vi "Read Friction Coefficient.vi"(8 "error in":errorcluster, 11 "Friction in":refnum<class "Friction.lvclass">) -> (0 "error out":errorcluster, 2 "Friction Coefficient":dbl, 3 "Friction out":refnum<class "Friction.lvclass">)   [LabVIEW 2016, in "Friction.lvclass"]
uses:
  Friction.lvclass
  Friction.lvclass/Friction.ctl
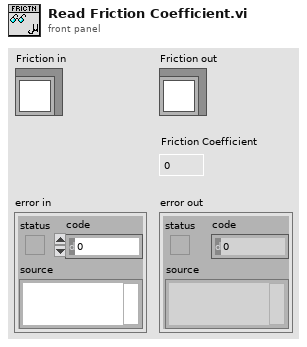
[diagram p1: front panel]
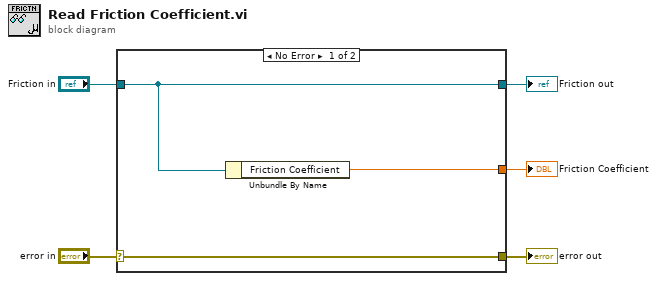
[diagram p0: block diagram]
diagram:
  n1 = case shown="No Error" "error in" {
    selector: "error in" -> [w8 w9]
    tunnel: [w8 w9] -> w4
    tunnel: [w7 w10] -> w2
    tunnel: "Friction in" -> [w7 w10]
    tunnel: [w6 _] -> w1
    frame No Error {
      n2 = Unbundle By Name(w7) -> ("Friction Coefficient"=w6:dbl)
    }
    frame Error {
    }
  }
  "error out" <- w4
  "Friction out" <- w2
  "Friction Coefficient" <- w1
